vi "Move Axis with Speed.vi"(8 "error in (no error)":errorcluster, 9 "Speed":dbl, 10 "Position":dbl, 11 "Axis":i32) -> (0 "error out":errorcluster)   [LabVIEW 2020, in "Manipulator CLI Driver.lvlib"]
uses:
  Manipulator CLI Driver.lvlib
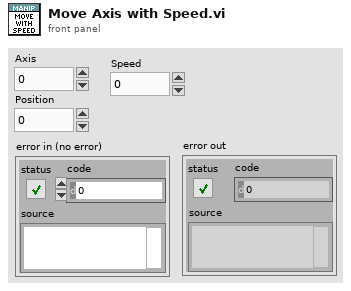
[diagram p1: front panel]
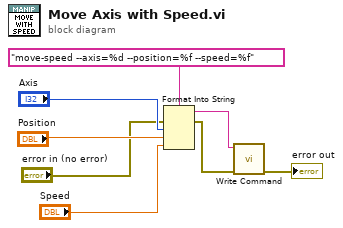
[diagram p0: block diagram]
diagram:
  n1 = Format Into String(format string="move-speed --axis=%d --position=%f --speed=%f", error in="error in (no error)", "Axis", "Position", "Speed") -> (resulting string=w4:string, error out=w2:errorcluster)  [unwired: 1 in]
  n2 = call "Write Command.vi"("error in (no error)"=w2, "command"=w4) -> ("error out"=→"error out":errorcluster)  [unwired: 7 in, 2 out]
